vi "Read Sensor Type.vi"(8 "error in (no error)":errorcluster, 10 "Node (3)":u8=3 caption="Node" min=3 max=128 step=1, 11 "VISA resource name":refnum<visa-resource-name>) -> (0 "error out":errorcluster, 1 "Sensor Type Name":string, 2 "Sensor Type Number":u32, 3 "VISA resource name out":refnum<visa-resource-name>)   [LabVIEW 2024, in "Bronkhorst FLOW-BUS.lvlib"]
doc: "Reads the value of the sensor type parameter that is used to select the proper set of units for a certain sensor.\n\nValid values are:\n0 = Pressure\n1 = Liquid volume\n2 = Liquid/gass mass\n3 = Gas volume\n4 = Other sensor type"
uses:
  Bronkhorst FLOW-BUS.lvlib
  Private/FLOW-BUS RW.ctl
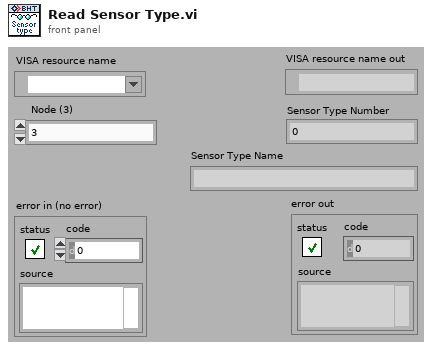
[diagram p1: front panel]
types:
  T1 = typedef "Bronkhorst FLOW-BUS.lvlib/FLOW-BUS RW.ctl" = cluster{"Node Address (3)":u8, "Communication Command":enum16{"Status message", "Send parameter with destination address and 00 response", "Send parameter with destination address", "Request parameter"}, "Process (0)":u16, "Parameter (0)":u16, "Data Type (0: Character)":enum16{"Character", "Integer", "Float or Long", "String"}, "Data for Char, Int, or Long (0)":u32, "Data for Float (0)":sgl, "Data for String":string, "Length of Requested String (0)":u8}
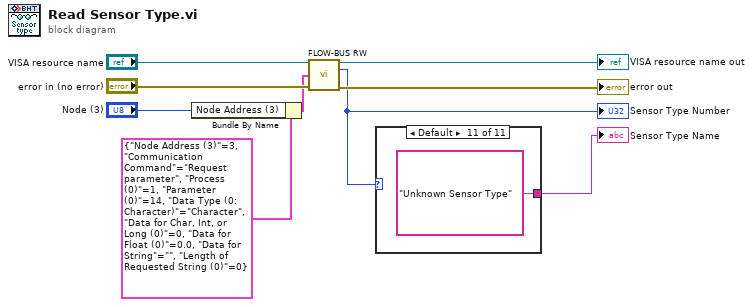
[diagram p0: block diagram]
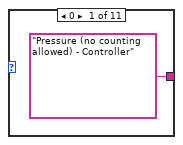
[diagram p2: hidden frame]
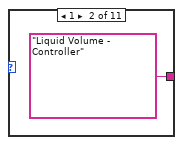
[diagram p3: hidden frame]
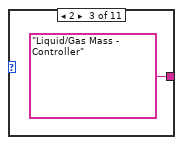
[diagram p4: hidden frame]
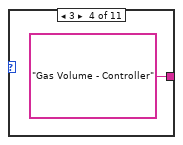
[diagram p5: hidden frame]
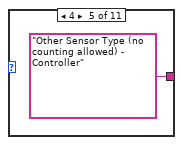
[diagram p6: hidden frame]
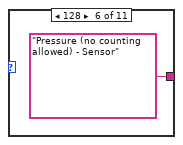
[diagram p7: hidden frame]
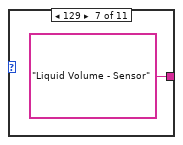
[diagram p8: hidden frame]
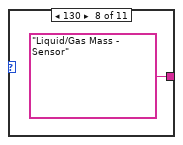
[diagram p9: hidden frame]
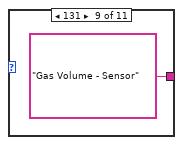
[diagram p10: hidden frame]
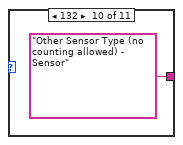
[diagram p11: hidden frame]
diagram:
  n1 = Bundle By Name(cluster=T1 {"Node Address (3)"=3, "Communication Command"=enum."Request parameter", "Process (0)"=1, "Parameter (0)"=14, "Data Type (0: Character)"=enum."Character", "Data for Char, Int, or Long (0)"=0, "Data for Float (0)"=0.0, "Data for String"="", "Length of Requested String (0)"=0} ("FLOW-BUS Command Settings"), "Node Address (3)"="Node (3)") -> (w2:T1)
  n2 = call "FLOW-BUS RW.vi"("VISA resource name"="VISA resource name", "FLOW-BUS Command Settings"=w2, "error in (no error)"="error in (no error)") -> ("VISA resource name out"=→"VISA resource name out":refnum<visa-resource-name>, "Requested Char, Int or Long"=w4:u32, "error out"=→"error out":errorcluster)  [unwired: 8 in, 2 out]
  "Sensor Type Number" <- w4
  n3 = case shown="Default" w4 {
    tunnel: ["Pressure (no counting allowed) - Controller" "Liquid Volume - Controller" "Liquid/Gas Mass - Controller" "Gas Volume - Controller" "Other Sensor Type (no counting allowed) - Controller" "Pressure (no counting allowed) - Sensor" "Liquid Volume - Sensor" "Liquid/Gas Mass - Sensor" "Gas Volume - Sensor" "Other Sensor Type (no counting allowed) - Sensor" "Unknown Sensor Type"] -> w3
    frame 0 {
    }
    frame 1 {
    }
    frame 2 {
    }
    frame 3 {
    }
    frame 4 {
    }
    frame 128 {
    }
    frame 129 {
    }
    frame 130 {
    }
    frame 131 {
    }
    frame 132 {
    }
    frame Default {
    }
  }
  "Sensor Type Name" <- w3
